vi "Select Worksheet.vi"   [LabVIEW 2013, in "XCel Report Engine.lvlib"]
doc: "Selects the active worksheet used by subsequent report operations.\n\nThis polymorphic VI provides instances for selecting a worksheet by name or by zero-based index.\n\nThe operation affects only the XCelReportEngine report session and does not require Microsoft Excel. An error is returned if the specified worksheet does not exist or the index is outside the valid range."
uses:
  XCel Report Engine.lvlib
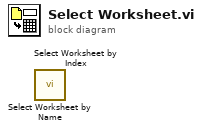
[diagram p0: block diagram]
diagram:
  n1 = call "Select Worksheet by Name.vi"() -> ()  [unwired: 3 in, 2 out]
  n2 = call "Select Worksheet by Index.vi"() -> ()  [unwired: 3 in, 2 out]
